vi "Close.vi"(8 "error in (no error)":errorcluster, 11 "Modbus PLC in":refnum<class "Modbus PLC.lvclass">) -> (0 "error out":errorcluster, 3 "Modbus PLC out":refnum<class "Modbus PLC.lvclass">)   [LabVIEW 2023, in "Modbus PLC.lvlib" / "Modbus PLC.lvclass"]
uses:
  Modbus PLC.lvclass
  Modbus PLC.lvclass/Modbus PLC.ctl
  <vilib>/NI/Modbus Library/API/Master/Modbus Master.lvclass
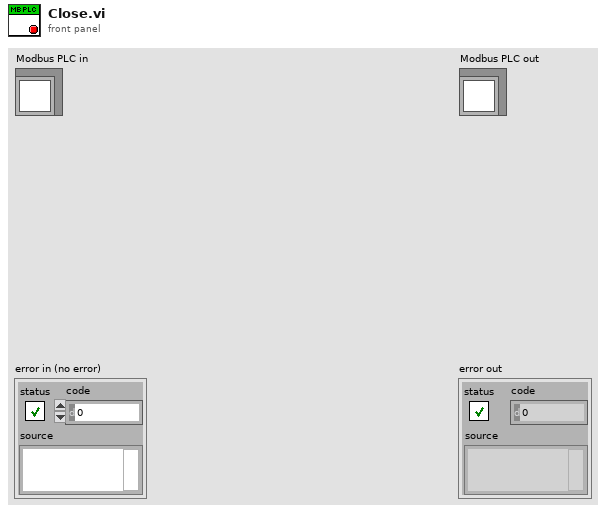
[diagram p1: front panel]
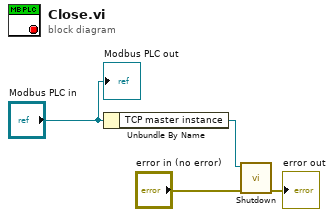
[diagram p0: block diagram]
diagram:
  n1 = Unbundle By Name("Modbus PLC in") -> ("TCP master instance"=w4:refnum<class "Modbus Master.lvclass">)
  n2 = call-dynamic "Shutdown.vi"("error in"="error in (no error)", "Modbus master in"=w4) -> ("error out"=→"error out":errorcluster)  [unwired: 9 in]
  "Modbus PLC out" <- "Modbus PLC in"
